vi "Write Topic.vi"(8 "error in (no error)":errorcluster, 10 "Topic":string, 11 "Process Object in":refnum<class "Process Object.lvclass">) -> (0 "error out":errorcluster, 3 "Process Object out":refnum<class "Process Object.lvclass">)   [LabVIEW 2015, in "Process Object.lvclass"]
uses:
  Process Object.lvclass
  Process Object.lvclass/Process Object.ctl
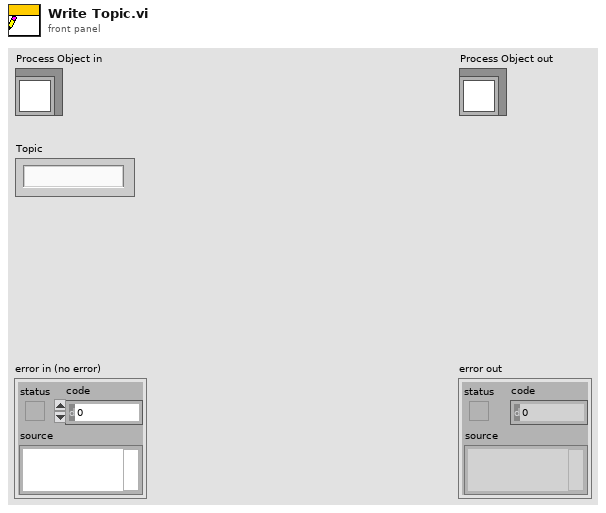
[diagram p1: front panel]
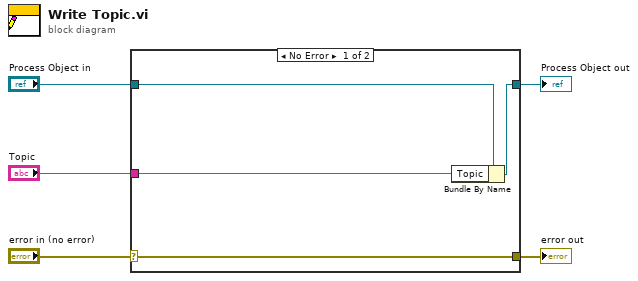
[diagram p0: block diagram]
diagram:
  n1 = case shown="No Error" "error in (no error)" {
    selector: "error in (no error)" -> [w9 w10]
    tunnel: [w9 w10] -> w4
    tunnel: [w7 w11] -> w2
    tunnel: "Process Object in" -> [w8 w11]
    tunnel: "Topic" -> [w6 _]
    frame No Error {
      n2 = Bundle By Name(cluster=w8, "Topic"=w6) -> (w7:refnum<class "Process Object.lvclass">)
    }
    frame Error {
    }
  }
  "error out" <- w4
  "Process Object out" <- w2
